vi "TrajectoryConfig_AddConstraints.vi"(9 "Constraints":variant[](array[variant]), 11 "inTRAJECTORY_CONFIG":T1 {"End Velocity" format="%20.4f"; "StartVelocity" format="%20.4f"; "Max Acceleration" format="%20.4f"; "MaxVelocity" format="%20.4f"}) -> (3 "outTRAJECTORY_CONFIG":T1 {"End Velocity" format="%20.4f"; "StartVelocity" format="%20.4f"; "Max Acceleration" format="%20.4f"; "MaxVelocity" format="%20.4f"})   [LabVIEW 2019, in "Trajectory_Library.lvlib"]
doc: "Add an array of constraints to this Trajectory Configuration\n\nParameters:\n - InTrajectoryConfig - The trajectory configuration data structure\n - Constraints -- Array of Trajectory constraint converted to a variant\n\nReturns:\n - OutTrajectoryConfig - Modified trajectory configuration data structure"
uses:
  Trajectory_Library.lvlib
  TypeDef/TRAJ_CONFIG.ctl
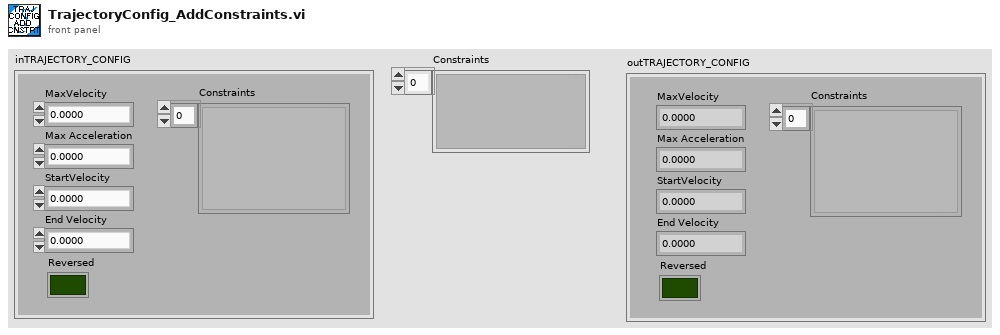
[diagram p1: front panel]
types:
  T1 = typedef "Trajectory_Library.lvlib/TRAJ_CONFIG.ctl" = cluster{"MaxVelocity":dbl, "Max Acceleration":dbl, "StartVelocity":dbl, "End Velocity":dbl, "Reversed":bool, "Constraints":variant[]}
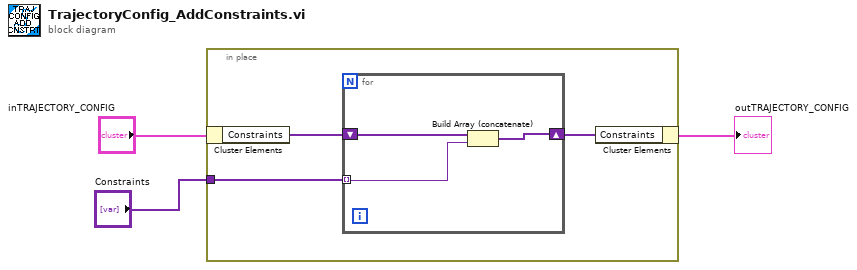
[diagram p0: block diagram]
diagram:
  n1 = in-place {
    in-place-border: "Constraints" -> [w6]
    n2 = in-place-cluster #1("inTRAJECTORY_CONFIG") -> ("Constraints"=w5:variant[])
    n3 = for {
      tunnel: w6 -> [w8] mode=indexing
      shift-right: [w7] -> w4
      shift-left: w5 -> [w9]
      n4 = Build Array (concatenate)(w9, w8) -> (w7:variant[])
    }
    n5 = in-place-cluster #1("Constraints"=w4) -> (→"outTRAJECTORY_CONFIG":T1)
  }
